vi "Save XML File.vi"(8 "error in":errorcluster, 10 "XML Configuration File Path":path=path "E:/Ballard - Arinc-429 CD/Example Database/Ballard/XML_000.XML", 11 "xml ref in":refnum<k24>) -> (0 "error out":errorcluster, 3 "xml ref out":refnum<k24>)   [LabVIEW 2020, in "Ballard_1553_Hardware_ni.lvlib"]
uses:
  Ballard_1553_Hardware_ni.lvlib
  C:/Users/Administrator/Desktop/GIT/Ballard-MIL-STD-1553-Custom-Device/Source/System Explorer/SubVIs/Parse XML Ballard/1.2/BTIXML_SerDes.dll
  Ballard-MIL-STD-1553-Custom-Device/Source/System Explorer/SubVIs/Parse XML Ballard/1.2/BTIXML_SerDes.dll
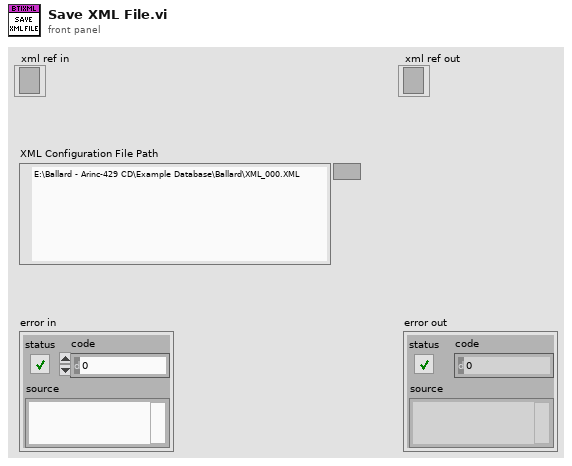
[diagram p1: front panel]
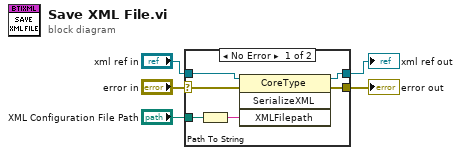
[diagram p0: block diagram]
diagram:
  n1 = case shown="No Error" "error in" {
    selector: "error in" -> [w6 w12]
    tunnel: "XML Configuration File Path" -> [w10 _]
    tunnel: [w9 w12] -> w4
    tunnel: [w8 w13] -> w3
    tunnel: "xml ref in" -> [w7 w13]
    frame No Error {
      n2 = Path To String(path=w10) -> (string=w11:string)
      n3 = invoke class="CoreType" method="SerializeXML"(reference=w7, error in=w6, "XMLFilepath"=w11) -> (reference out=w8:refnum<k24>, error out=w9:errorcluster)  [unwired: 1 in, 2 out]
    }
    frame Error {
    }
  }
  "error out" <- w4
  "xml ref out" <- w3
